vi "Untitled 1.vi"() -> ()   [LabVIEW 2018]
uses:
  <vilib>/Instr/_visa.llb/VISA Configure Serial Port (Instr).vi
panel:
  in  "stop 2":bool
  in  "Boolean":bool
  out "read buffer":string
  in  "VISA resource name":refnum<visa-resource-name>
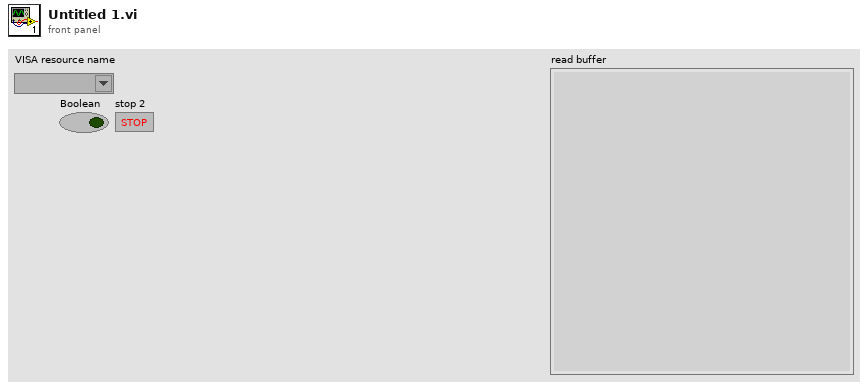
[diagram p1: front panel]
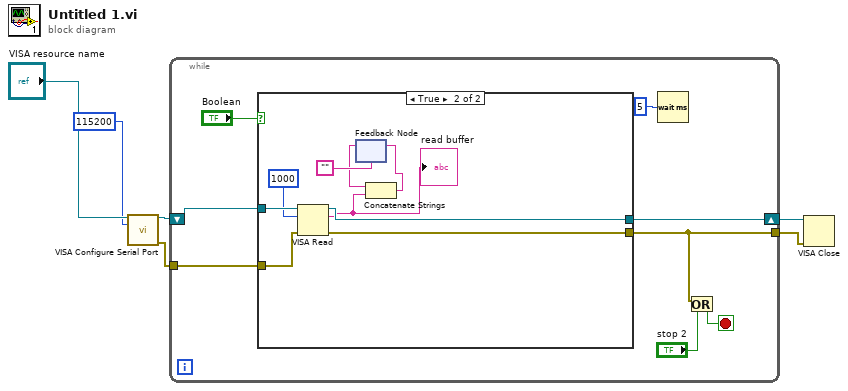
[diagram p0: block diagram]
diagram:
  n1 = call-poly "VISA Configure Serial Port"("VISA resource name"="VISA resource name", "baud rate (9600)"=u32 115200) -> ("VISA resource name out"=w4:refnum<visa-resource-name>, "error out"=w3:errorcluster)  [unwired: 12 in]
  n2 = while {
    tunnel: w3 -> [w10]
    tunnel: [w8] -> w1
    shift-right: [w11] -> w2
    shift-left: w4 -> [w12]
    stop <- w9 stop-if-true
    n3 = case shown="True" "Boolean" {
      tunnel: w12 -> [w16 w25]
      tunnel: [w16 w24] -> w11
      tunnel: [w15 w23] -> w8
      tunnel: w10 -> [w15 w22]
      frame False {
      }
      frame True {
        n4 = VISA Read(VISA resource name=w25, byte count=u32 1000, error in (no error)=w22) -> (VISA resource name out=w24:refnum<visa-resource-name>, read buffer=w17:string, error out=w23:errorcluster)  [unwired: 1 out]
        "read buffer" <- w17
        n5 = feedback #1("") -> (w20:string)
        n6 = Concatenate Strings(w20, w17) -> (w19:string)
        n7 = feedback-in #1(w19) -> ()
      }
    }
    n8 = Wait (ms)(milliseconds to wait=u32 5) -> ()  [unwired: 1 out]
    n9 = Or(x=w8, y="stop 2") -> (x .or. y?=w9:bool)
  }
  n10 = VISA Close(VISA resource name=w2, error in (no error)=w1) -> ()  [unwired: 1 out]
